vi "grape test.vi"() -> ()   [LabVIEW 2010]
panel:
  out "Waveform Chart":dbl[](graph)
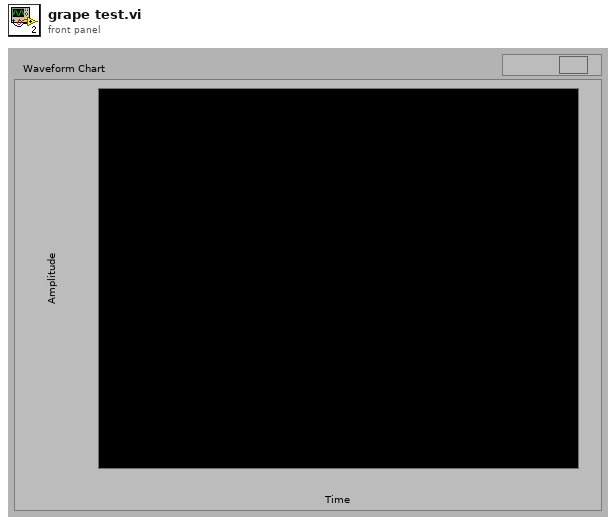
[diagram p1: front panel]
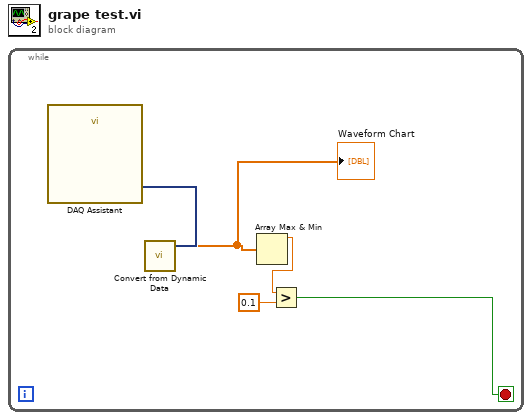
[diagram p0: block diagram]
diagram:
  n1 = while {
    stop <- w4 stop-if-true
    n2 = call "DAQ Assistant"() -> ("data"=w3:dynamicdata)  [unwired: 16 in, 3 out]
    n3 = call "Convert from Dynamic Data"("Dynamic Data Type"=w3) -> ("Array"=w1:dbl[])  [unwired: 3 in]
    "Waveform Chart" <- w1
    n4 = Array Max & Min(array=w1) -> (max value=w2:dbl)  [unwired: 3 out]
    n5 = Greater?(x=w2, y=0.1) -> (0:w4:bool)
  }
